vi "SubtractZeroes.vi"(7 "NoiseFloorValue (Pressure Units)":dbl=0.2, 10 "RawPressure":dbl[][](array[numeric]), 11 "Zeroes":dbl[](array[numeric])) -> (1 "AdequatedP?":bool[](array[boolean]), 2 "MaxdP":dbl[](array[numeric]), 3 "ZeroedPressure":dbl[][](array[numeric]))   [LabVIEW 2013]
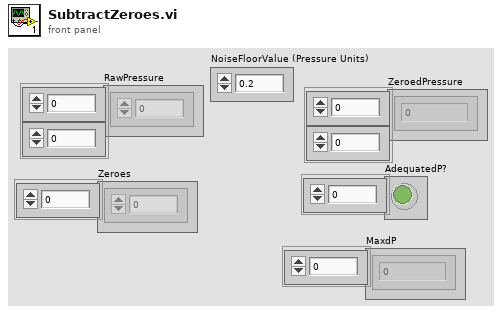
[diagram p1: front panel]
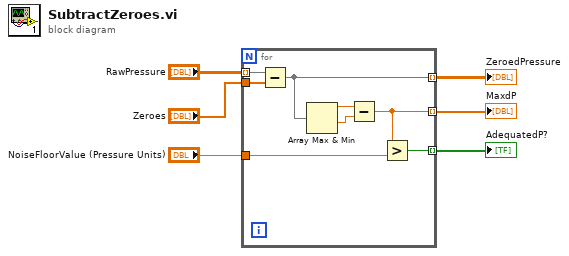
[diagram p0: block diagram]
diagram:
  n1 = for {
    tunnel: [w12] -> w4 mode=indexing
    tunnel: "RawPressure" -> [w14] mode=indexing
    tunnel: "Zeroes" -> [w13]
    tunnel: "NoiseFloorValue (Pressure Units)" -> [w9]
    tunnel: [w8] -> w2 mode=indexing
    tunnel: [w7] -> w1 mode=indexing
    n2 = Subtract(x=w14, y=w13) -> (x-y=w12:dbl[])
    n3 = Array Max & Min(array=w12) -> (max value=w11:dbl, min value=w10:dbl)  [unwired: 2 out]
    n4 = Subtract(x=w11, y=w10) -> (x-y=w7:dbl)
    n5 = Greater?(x=w7, y=w9) -> (0:w8:bool)
  }
  "ZeroedPressure" <- w4
  "AdequatedP?" <- w2
  "MaxdP" <- w1
